vi "Construct ModelLaunchesActor.vi"(10 "Actor to Launch":refnum<class "Actor.lvclass">, 11 "Auto-Launch Nested Models":refnum<class "IModel.lvclass">[](array[class])) -> (3 "ModelLaunchesActor out":refnum<class "ModelLaunchesActor.lvclass">)   [LabVIEW 2017, in "ModelLaunchesActor.lvclass"]
uses:
  ModelLaunchesActor.lvclass
  C:/Git/mva-core/Source/IModel/IModel/IModel.lvclass
  <vilib>/ActorFramework/Actor/Actor.lvclass
  Source/IModel/IModel/IModel.lvclass
  Source/IModel/IModel/IModel.lvclass/IModel.ctl
  ModelLaunchesActor.lvclass/ModelLaunchesActor.ctl
  Source/IModel/IModel Messages/Auto-Launch Models Msg/Pack Auto-Launch Models Msg.vi
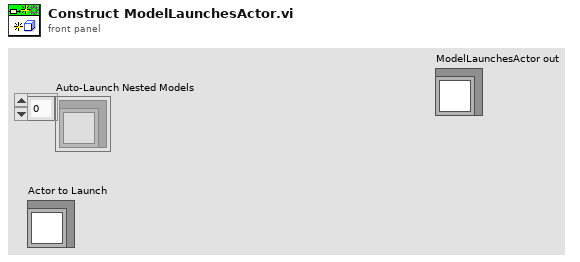
[diagram p1: front panel]
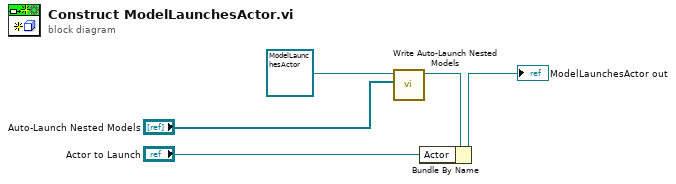
[diagram p0: block diagram]
diagram:
  n1 = call "Write Auto-Launch Nested Models.vi"("Auto-Launch Nested Models"="Auto-Launch Nested Models", "IModel In"=refnum<class "ModelLaunchesActor.lvclass"> refnum ("ModelLaunchesActor in")) -> ("IModel Out"=w2:refnum<class "ModelLaunchesActor.lvclass">)  [unwired: 9 in]
  n2 = Bundle By Name(cluster=w2, "Actor"="Actor to Launch") -> (→"ModelLaunchesActor out":refnum<class "ModelLaunchesActor.lvclass">)
